vi "GetTandH.vi"(8 "error in (no error)":errorcluster, 11 "Instrument.Temperhum in":refnum<class "Instrument.Temperhum.lvclass">) -> (0 "error out":errorcluster, 1 "Humidity (%RH)":dbl, 2 "Temperature (K)":dbl, 3 "Instrument.Temperhum out":refnum<class "Instrument.Temperhum.lvclass">)   [LabVIEW 2019, in "Instrument.Temperhum.lvclass"]
uses:
  Instrument.Temperhum.lvclass
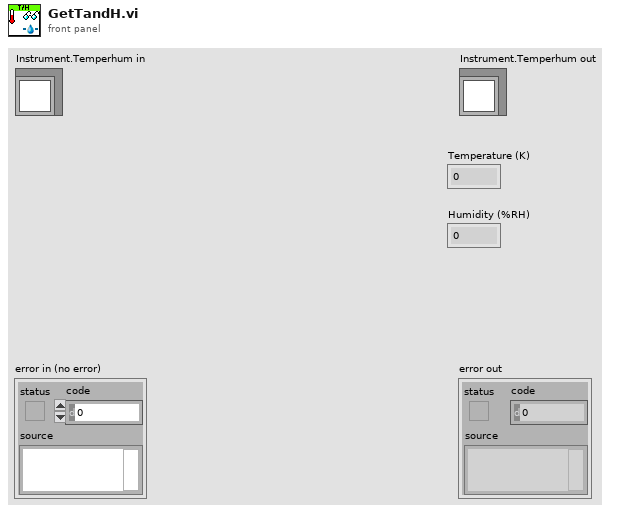
[diagram p1: front panel]
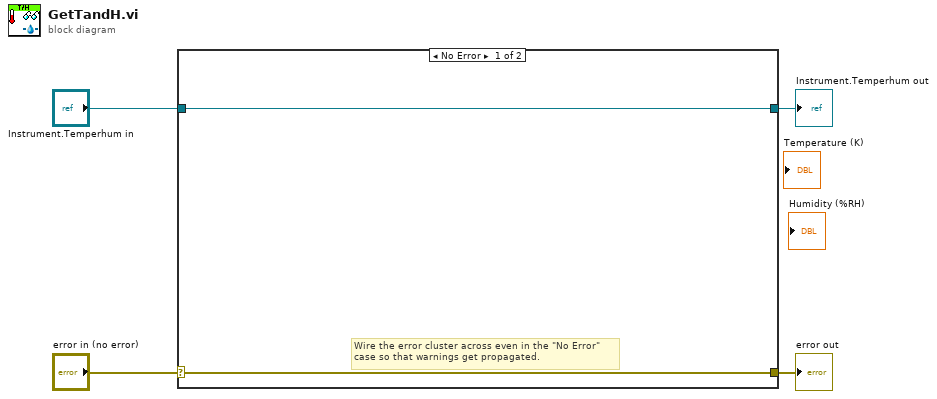
[diagram p0: block diagram]
diagram:
  n1 = case shown="No Error" "error in (no error)" {
    selector: "error in (no error)" -> [w5 w8]
    tunnel: [w5 w8] -> w3
    tunnel: [w6 w7] -> w1
    tunnel: "Instrument.Temperhum in" -> [w6 w7]
    frame No Error {
      # "Wire the error cluster across even in the \"No Error\"\ncase so that warnings get propagated."
    }
    frame Error {
    }
  }
  "error out" <- w3
  "Instrument.Temperhum out" <- w1
